vi "D012L_Motors.vi"() -> ()   [LabVIEW 2011]
uses:
  PIMotorController.llb/PI_Axis.ctl
panel:
  in  "PI Axis info":T2={"Piezo X"={"System #"=0, "Axis ID"="", "Multiplier"=1.0}, "Piezo Y"={"System #"=0, "Axis ID"="", "Multiplier"=1.0}, "Piezo Z"={"System #"=0, "Axis ID"="0", "Multiplier"=1.0}, "Magnet Z"={"System #"=0, "Axis ID"="0", "Multiplier"=1.0}, "Magnet Rotation"={"System #"=0, "Axis ID"="0", "Multiplier"=1.0}, "Objective X"={"System #"=0, "Axis ID"="", "Multiplier"=1.0}, "Objective Y"={"System #"=0, "Axis ID"="", "Multiplier"=1.0}}
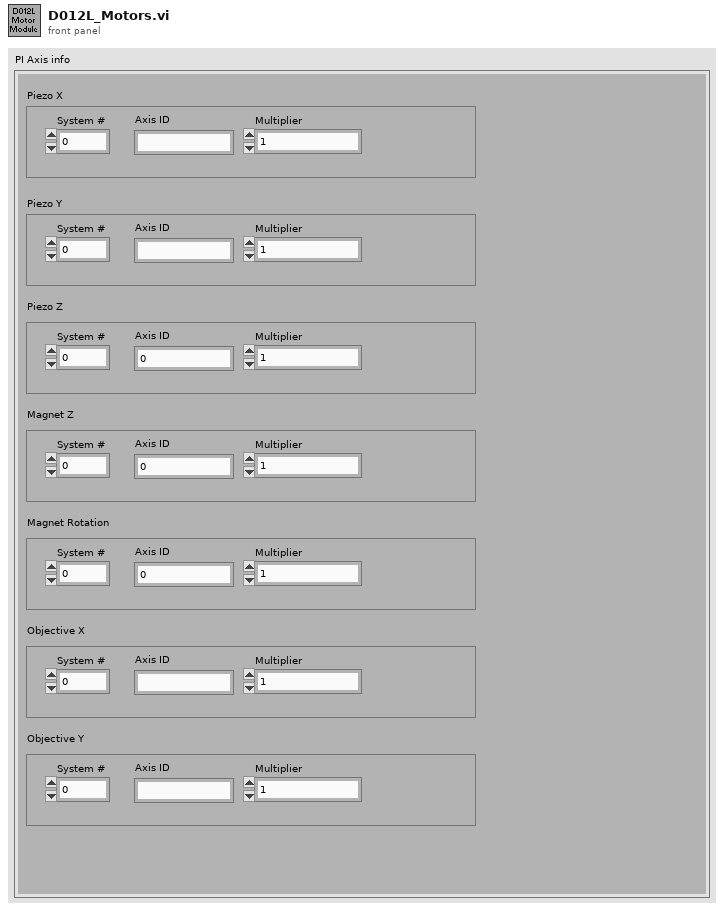
[diagram p1: front panel]
types:
  T1 = typedef "PI_Axis.ctl" = cluster{"System #":i32, "Axis ID":string, "Multiplier":dbl}
  T2 = cluster{"Piezo X":T1, "Piezo Y":T1, "Piezo Z":T1, "Magnet Z":T1, "Magnet Rotation":T1, "Objective X":T1, "Objective Y":T1}
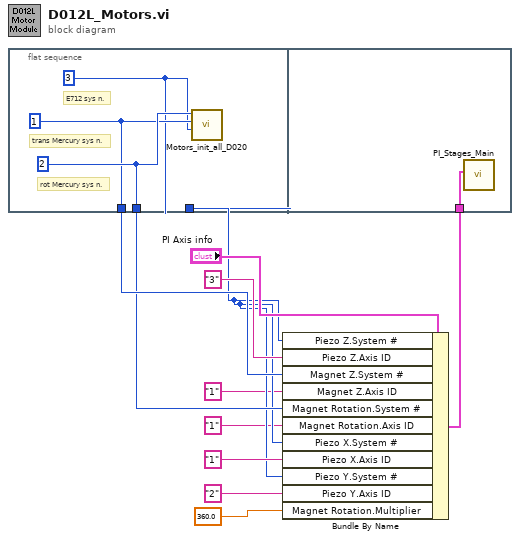
[diagram p0: block diagram]
diagram:
  n1 = flat-sequence {
    tunnel: [w13] -> w9
    tunnel: [w14] -> w8
    tunnel: [w12] -> w4
    tunnel: w10 -> [w15]
    frame #0 {
      w13 = 1 ("Mercury System no.")
      w12 = 3 ("E712 System no.")
      w14 = 2 ("Mercury System no.")
      # "trans Mercury sys n."
      # "E712 sys n."
      # "rot Mercury sys n."
      n2 = call "Motors_init_all_D020.vi"("Mercury Rotation"=w14, "Mercury Translation"=w13, "E712 System no."=w12) -> ()  [unwired: 4 in]
    }
    frame #1 {
      n3 = call "PI_Stages_Main.vi"("PI Axis info"=w15) -> ()  [unwired: 11 in]
    }
  }
  n4 = Bundle By Name(cluster="PI Axis info", "Piezo Z.System #"=w4, "Piezo Z.Axis ID"="3", "Magnet Z.System #"=w9, "Magnet Z.Axis ID"="1", "Magnet Rotation.System #"=w8, "Magnet Rotation.Axis ID"="1", "Piezo X.System #"=w4, "Piezo X.Axis ID"="1", "Piezo Y.System #"=w4, "Piezo Y.Axis ID"="2", "Magnet Rotation.Multiplier"=360.0) -> (w10:T2)
